vi "CRYOptions.vi"() -> ()   [LabVIEW 2013]
panel:
  in  "A&R option":bool=TRUE
  in  "Loudness rating":bool=TRUE
  in  "RTA option":bool=TRUE
  in  "FFT option":bool=TRUE
  in  "TSR option":bool=TRUE
  in  "Distortion":bool=TRUE
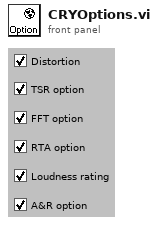
[diagram p1: front panel]
diagram:
